vi "Zero Actuator.vi"() -> ()   [LabVIEW 2012]
uses:
  Controls/Zero Actuator Shifter.ctl
  <vilib>/Rock Robotics/WPI/Joystick/WPI_JoystickGetSetRefNum.vi
  Globals/Potentiometers.vi
  Globals/Are We Calibrating Actuator.vi
  Globals/Jaguar Commands.vi
  <vilib>/Utility/file.llb/Write To Spreadsheet File (DBL).vi
  Globals/Actuator Home Position.vi
  Globals/Max Tipper Angle.vi
panel:
  in  "Previous Volt Limit":dbl
  in  "F. Bumper Pos.":dbl
  out "State":T1
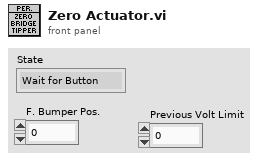
[diagram p1: front panel]
types:
  T1 = typedef "Zero Actuator Shifter.ctl" = enum16{"Wait for Button", "Move to Front", "Move to Back", "Set Home"}
  T2 = typedef "WPI_JoystickDevRef.ctl" = cluster{"Device":T3}
  T3 = typedef "WPI_JoystickDeviceEnum.ctl" = enum16{"USB 1", "USB 2", "USB 3", "USB 4", "Kinect 1", "Kinect 2"}
  T4 = typedef "WPI_AnalogChannelDevRef.ctl" = cluster{"DevStatus":errorcluster, "Analog Module":T5, "Analog Channel":T6}
  T5 = typedef "FPGA_TypedefAnalogModule.ctl" = enum16{"Analog Module 1", "Analog Module 2"}
  T6 = typedef "FPGA_AIChannel.ctl" = enum8{"AI 1", "AI 2", "AI 3", "AI 4", "AI 5", "AI 6", "AI 7", "AI 8", "Invalid"}
  T7 = cluster{"Front Left":T4, "Front Right":T4, "Rear Left":T4, "Rear Right":T4, "Actuator":T4}
  T8 = typedef "WPI_JoystickButtonState.ctl" = cluster{"Button 1":bool, "Button 2":bool, "Button 3":bool, "Button 4":bool, "Button 5":bool, "Button 6":bool, "Button 7":bool, "Button 8":bool, "Button 9":bool, "Button 10":bool, "Button 11":bool, "Button 12":bool}
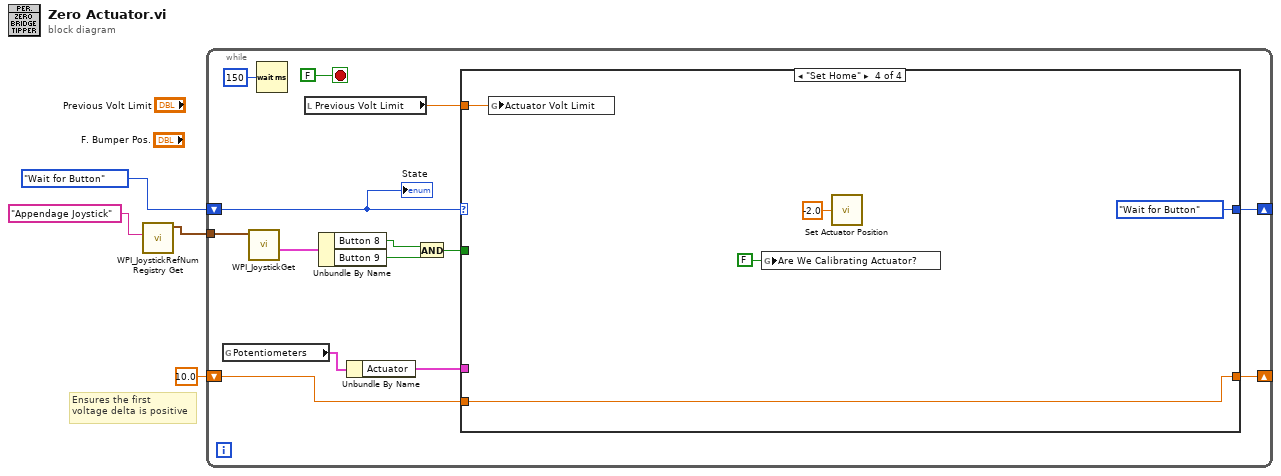
[diagram p0: block diagram]
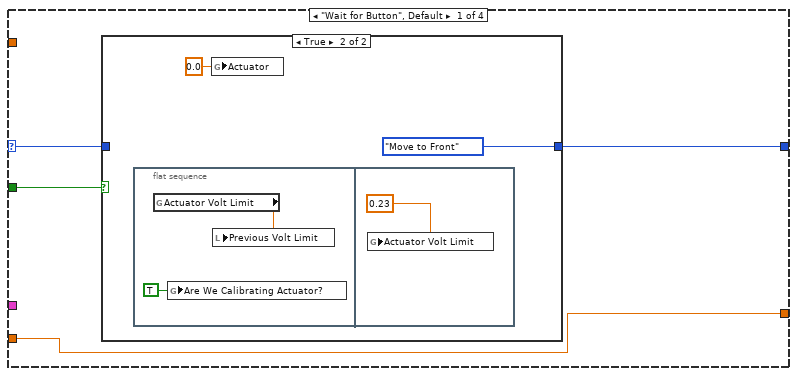
[diagram p2: hidden frame]
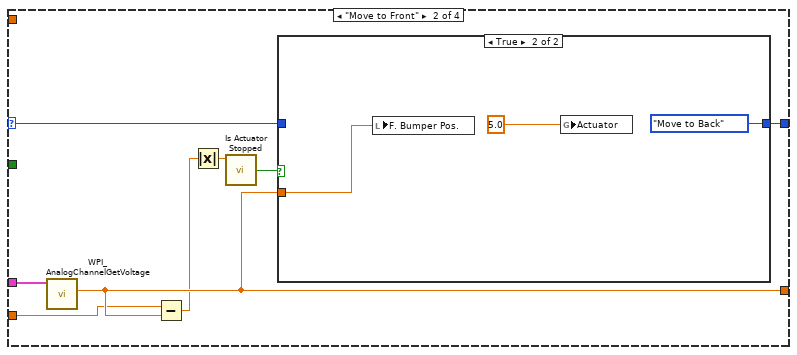
[diagram p4: hidden frame]
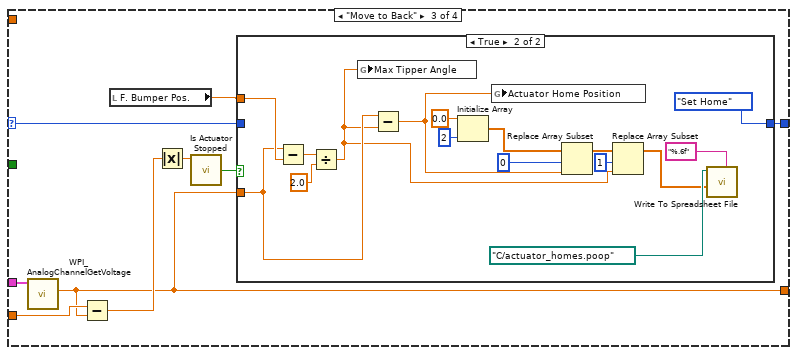
[diagram p6: hidden frame]
diagram:
  # "Ensures the first\nvoltage delta is positive"
  n1 = call <vilib>:"WPI_JoystickRefNum Registry Get.vi"("refnum name"="Appendage Joystick") -> ("JoystickDevRef"=w4:T2)  [unwired: 1 in, 9 out]
  n2 = while {
    tunnel: w4 -> [w15]
    shift-right: [w13] -> _
    shift-left: Zero_Actuator_Shifter."Wait for Button" ("States") -> [w12]
    shift-right: [w10] -> _
    shift-left: 10.0 ("Voltage") -> [w9]
    stop <- FALSE stop-if-true
    n3 = global read "Potentiometers.vi" "Potentiometers"() -> (w14:T7)
    n4 = call <vilib>:"WPI_JoystickGet.vi"("JoystickDevRef"=w15) -> ("Buttons"=w16:T8)  [unwired: 4 in, 2 out]
    n5 = Wait (ms)(milliseconds to wait=u32 150) -> ()  [unwired: 1 out]
    n6 = local read "Previous Volt Limit"() -> (w5:dbl)
    n7 = Unbundle By Name(w16) -> ("Button 8"=w8:bool, "Button 9"=w7:bool)
    n8 = Unbundle By Name(w14) -> ("Actuator"=w11:T4)
    n9 = And(x=w8, y=w7) -> (x .and. y?=w6:bool)
    n10 = case shown="\"Set Home\"" w12 {
      selector: w12 -> [w20 w35 w46 _]
      tunnel: [w21 w34 w43 Zero_Actuator_Shifter."Wait for Button" ("States")] -> w13
      tunnel: w6 -> [w22 _ _ _]
      tunnel: w11 -> [_ w36 w45 _]
      tunnel: [w19 w33 w42 w71] -> w10
      tunnel: w9 -> [w19 w32 w44 w71]
      tunnel: w5 -> [_ _ _ w67]
      frame "Wait for Button", Default {
        n11 = case shown="True" w22 {
          tunnel: [w23 Zero_Actuator_Shifter."Move to Front" ("States")] -> w21
          tunnel: w20 -> [w23 _]
          frame False {
          }
          frame True {
            n12 = flat-sequence {
              frame #0 {
                n13 = global read "Jaguar Commands.vi" "Actuator Volt Limit"() -> (w27:dbl)
                n14 = global write "Are We Calibrating Actuator.vi" "Are We Calibrating Actuator?"(TRUE ("Are We Calibrating Actuator?")) -> ()
                n15 = local write "Previous Volt Limit"(w27) -> ()
              }
              frame #1 {
                n16 = global write "Jaguar Commands.vi" "Actuator Volt Limit"(0.23) -> ()
              }
            }
            n17 = global write "Jaguar Commands.vi" "Actuator"(0.0 ("Actuator")) -> ()
          }
        }
      }
      frame "Move to Front" {
        n18 = call <vilib>:"WPI_AnalogChannelGetVoltage.vi"("AIDeviceRef"=w36) -> ("Voltage"=w33:dbl)  [unwired: 8 in, 2 out]
        n19 = Subtract(x=w32, y=w33) -> (x-y=w31:dbl)
        n20 = Absolute Value(x=w31) -> (abs(x)=w29:dbl)
        n21 = call "Is Actuator Stopped.vi"("Voltage Delta"=w29) -> ("Stopped?"=w30:bool)  [unwired: 1 in]
        n22 = case shown="True" w30 {
          tunnel: w33 -> [_ w38]
          tunnel: w35 -> [w37 _]
          tunnel: [w37 Zero_Actuator_Shifter."Move to Back" ("States")] -> w34
          frame False {
          }
          frame True {
            n23 = local write "F. Bumper Pos."(w38) -> ()
            n24 = global write "Jaguar Commands.vi" "Actuator"(5.0 ("Actuator")) -> ()
          }
        }
      }
      frame "Move to Back" {
        n25 = call <vilib>:"WPI_AnalogChannelGetVoltage.vi"("AIDeviceRef"=w45) -> ("Voltage"=w42:dbl)  [unwired: 8 in, 2 out]
        n26 = Subtract(x=w44, y=w42) -> (x-y=w49:dbl)
        n27 = local read "F. Bumper Pos."() -> (w41:dbl)
        n28 = Absolute Value(x=w49) -> (abs(x)=w47:dbl)
        n29 = call "Is Actuator Stopped.vi"("Voltage Delta"=w47) -> ("Stopped?"=w48:bool)  [unwired: 1 in]
        n30 = case shown="True" w48 {
          tunnel: w42 -> [_ w59]
          tunnel: w46 -> [w50 _]
          tunnel: [w50 Zero_Actuator_Shifter."Set Home" ("States")] -> w43
          tunnel: w41 -> [_ w62]
          frame False {
          }
          frame True {
            n31 = Subtract(x=w59, y=w62) -> (x-y=w61:dbl)
            n32 = Divide(x=w61, y=2.0) -> (x/y=w55:dbl)
            n33 = global write "Max Tipper Angle.vi" "Max Tipper Angle"(w55) -> ()
            n34 = Subtract(x=w59, y=w55) -> (x-y=w54:dbl)
            n35 = Initialize Array(0.0 ("element"), 2 ("dimension size")) -> (w56:dbl[])
            n36 = global write "Actuator Home Position.vi" "Actuator Home Position"(w54) -> ()
            n37 = Replace Array Subset(array=w56, new element=w54, index=0) -> (w52:dbl[])
            n38 = Replace Array Subset(array=w52, new element=w55, index=1) -> (w51:dbl[])
            n39 = call-poly <vilib>:"Write To Spreadsheet File.vi"("format (%.3f)"="%.6f", "1D data"=w51, "file path (dialog if empty)"=path "C:/actuator_homes.poop") -> ()  [unwired: 5 in, 1 out]
          }
        }
      }
      frame "Set Home" {
        n40 = global write "Jaguar Commands.vi" "Actuator Volt Limit"(w67) -> ()
        n41 = global write "Are We Calibrating Actuator.vi" "Are We Calibrating Actuator?"(FALSE ("Are We Calibrating Actuator?")) -> ()
        n42 = call "Set Actuator Position.vi"("Setpoint from Home"=-2.0) -> ()
      }
    }
    "State" <- w12
  }
